vi "Auto Roller Logic.vi"(10 "chambering speed":dbl=0.55, 11 "intake speed":dbl=1.0) -> (3 "ok":bool)   [LabVIEW 2011]
panel:
  in  "Delay (ms)":u32=500
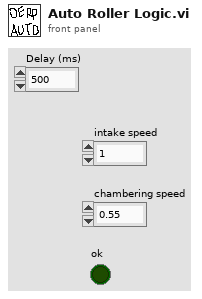
[diagram p1: front panel]
types:
  T1 = enum16{"Intake", "Chambering Front", "Chambering Rear"}
  T2 = typedef "WPI_DigitalInputDevRef.ctl" = cluster{"DevStatus":errorcluster, "DIO Channel":T3, "Digital Module":T4}
  T3 = typedef "FPGA_DIOChannel.ctl" = enum8{"DIO 1", "DIO 2", "DIO 3", "DIO 4", "DIO 5", "DIO 6", "DIO 7", "DIO 8", "DIO 9", "DIO 10", "DIO 11", "DIO 12", "DIO 13", "DIO 14", "Invalid"}
  T4 = typedef "FPGA_TypedefDigitalModule.ctl" = enum16{"Digital Module 1", "Digital Module 2"}
  T5 = typedef "WPI_MotorControlDeviceRef.ctl" = cluster{"DeviceStatus":errorcluster, "Type":enum16{"PWM", "CAN"}, "PWM":cluster{"Digital Module":T4, "PWM Channel":T6, "DeadBand":T7}, "CAN":cluster{"Device Number":u8, "Control Mode":T8, "Semaphore":T9, "Max Vout":dbl}, "Invert":bool, "TransformRef":T10, "InvTransformRef":T10}
  T6 = typedef "FPGA_DIOPWMChannel.ctl" = enum8{"PWM 1", "PWM 2", "PWM 3", "PWM 4", "PWM 5", "PWM 6", "PWM 7", "PWM 8", "PWM 9", "PWM 10", "Invalid"}
  T7 = typedef "WPI_PWMDeadband.ctl" = cluster{"Name":string, "maxPositivePwm":i32, "minPositivePwm":i32, "centerPwm":i32, "maxNegativePwm":i32, "minNegativePwm":i32, "angularRange":u16}
  T8 = typedef "WPI_CANJaguar_ControlMode.ctl" = enum8{"Percent VBus", "Current", "Speed", "Position", "Voltage"}
  T9 = typedef "Semaphore RefNum" = refnum<k1>
  T10 = typedef "WPI_PWMTransform_ConPane.ctl" = refnum<vi>
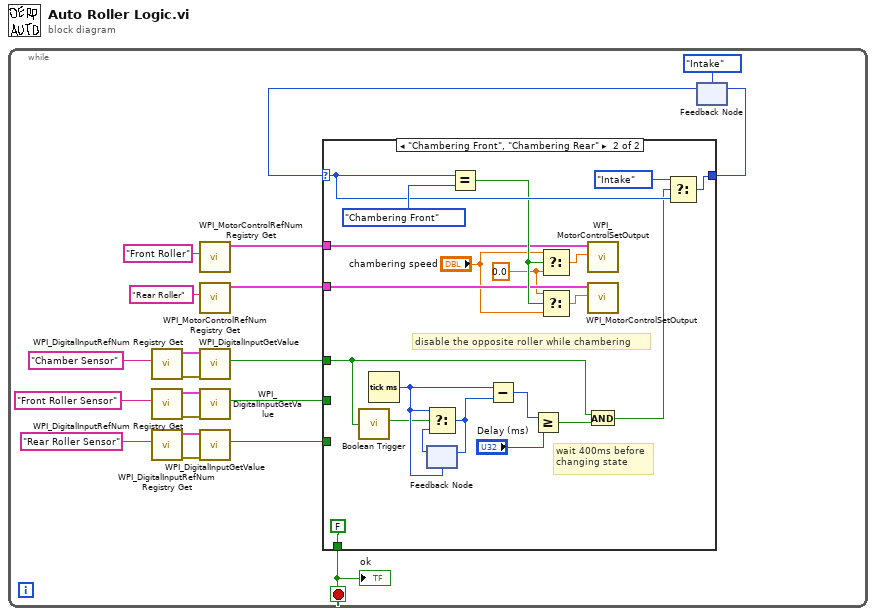
[diagram p0: block diagram]
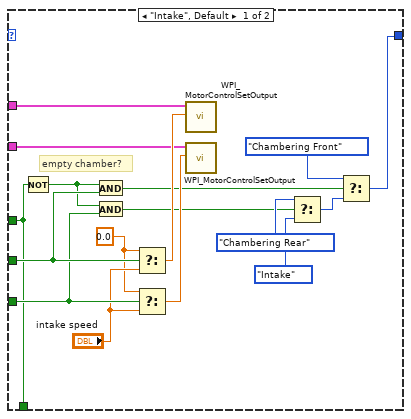
[diagram p2: hidden frame]
diagram:
  n1 = while {
    stop <- w1 stop-if-true
    n2 = call <vilib>:"WPI_DigitalInputRefNum Registry Get.vi"("refnum name"="Chamber Sensor") -> ("error out"=w18:errorcluster, "DigitalInputDevRef"=w19:T2)  [unwired: 9 in]
    n3 = call <vilib>:"WPI_DigitalInputRefNum Registry Get.vi"("refnum name"="Front Roller Sensor") -> ("error out"=w17:errorcluster, "DigitalInputDevRef"=w16:T2)  [unwired: 9 in]
    n4 = call <vilib>:"WPI_DigitalInputRefNum Registry Get.vi"("refnum name"="Rear Roller Sensor") -> ("error out"=w12:errorcluster, "DigitalInputDevRef"=w13:T2)  [unwired: 9 in]
    n5 = call <vilib>:"WPI_MotorControlRefNum Registry Get.vi"("refnum name"="Front Roller") -> ("MotorControlDevRef"=w9:T5)  [unwired: 9 in, 1 out]
    n6 = call <vilib>:"WPI_MotorControlRefNum Registry Get.vi"("refnum name"="Rear Roller") -> ("MotorControlDevRef"=w8:T5)  [unwired: 9 in, 1 out]
    n7 = call <vilib>:"WPI_DigitalInputGetValue.vi"("error in (no error)"=w18, "DigitalInputDevRef"=w19) -> ("Value"=w2:bool)  [unwired: 7 in, 2 out]
    n8 = call <vilib>:"WPI_DigitalInputGetValue.vi"("error in (no error)"=w17, "DigitalInputDevRef"=w16) -> ("Value"=w4:bool)  [unwired: 7 in, 2 out]
    n9 = call <vilib>:"WPI_DigitalInputGetValue.vi"("error in (no error)"=w12, "DigitalInputDevRef"=w13) -> ("Value"=w3:bool)  [unwired: 7 in, 2 out]
    n10 = feedback #1(T1."Intake") -> (w7:T1)
    n11 = case shown="\"Chambering Front\", \"Chambering Rear\"" w7 {
      selector: w7 -> [_ w57]
      tunnel: w4 -> [w30 _]
      tunnel: w9 -> [w25 w50]
      tunnel: w3 -> [w27 _]
      tunnel: w8 -> [w24 w51]
      tunnel: [w35 w56] -> w6
      tunnel: w2 -> [w21 w41]
      tunnel: [w21 FALSE] -> w1
      frame "Intake", Default {
        w22 = 0.0 ("t")
        # "empty chamber?"
        n12 = Not(x=w21) -> (.not. x?=w26:bool)
        n13 = And(x=w26, y=w30) -> (x .and. y?=w29:bool)
        n14 = And(x=w26, y=w27) -> (x .and. y?=w28:bool)
        n15 = Select(t=w22, s=w30, f="intake speed") -> (s? t:f=w37:dbl)
        n16 = Select(t=w22, s=w27, f="intake speed") -> (s? t:f=w36:dbl)
        n17 = call <vilib>:"WPI_MotorControlSetOutput.vi"("Output"=w37, "MotorControlDevRef"=w25) -> ()  [unwired: 8 in, 2 out]
        n18 = call <vilib>:"WPI_MotorControlSetOutput.vi"("Output"=w36, "MotorControlDevRef"=w24) -> ()  [unwired: 8 in, 2 out]
        n19 = Select(t=T1."Chambering Rear", s=w28, f=T1."Intake") -> (s? t:f=w33:T1)
        n20 = Select(t=T1."Chambering Front", s=w29, f=w33) -> (s? t:f=w35:T1)
      }
      frame "Chambering Front", "Chambering Rear" {
        w48 = 0.0 ("f")
        # "wait 400ms before\nchanging state"
        # "disable the opposite roller while chambering"
        n21 = call "Boolean Trigger.vi"("input"=w41) -> ("rising edge"=w42:bool)  [unwired: 2 in, 1 out]
        n22 = Tick Count (ms)() -> (millisecond timer value=w44:u32)
        n23 = feedback #2(w44) -> (w43:u32)
        n24 = Select(t=w44, s=w42, f=w43) -> (s? t:f=w45:u32)
        n25 = feedback-in #2(w45) -> ()
        n26 = Equal?(x=w57, y=T1."Chambering Front") -> (x = y?=w52:bool)
        n27 = Subtract(x=w44, y=w45) -> (x-y=w46:u32)
        n28 = Greater Or Equal?(x=w46, y="Delay (ms)") -> (x >= y?=w47:bool)
        n29 = Select(t="chambering speed", s=w52, f=w48) -> (s? t:f=w54:dbl)
        n30 = Select(t=w48, s=w52, f="chambering speed") -> (s? t:f=w53:dbl)
        n31 = call <vilib>:"WPI_MotorControlSetOutput.vi"("Output"=w54, "MotorControlDevRef"=w50) -> ()  [unwired: 8 in, 2 out]
        n32 = call <vilib>:"WPI_MotorControlSetOutput.vi"("Output"=w53, "MotorControlDevRef"=w51) -> ()  [unwired: 8 in, 2 out]
        n33 = And(x=w41, y=w47) -> (x .and. y?=w40:bool)
        n34 = Select(t=T1."Intake", s=w40, f=w57) -> (s? t:f=w56:T1)
      }
    }
    "ok" <- w1
    n35 = feedback-in #1(w6) -> ()
  }
